vi "Red_Micro_Parse.vi"(10 "Data":string, 11 "String Array In":string[](array[string])) -> (2 "Redundant Micro out":T1, 3 "String Array Out":string[](array[string]))   [LabVIEW 2021]
uses:
  type defs/Redundant.ctl
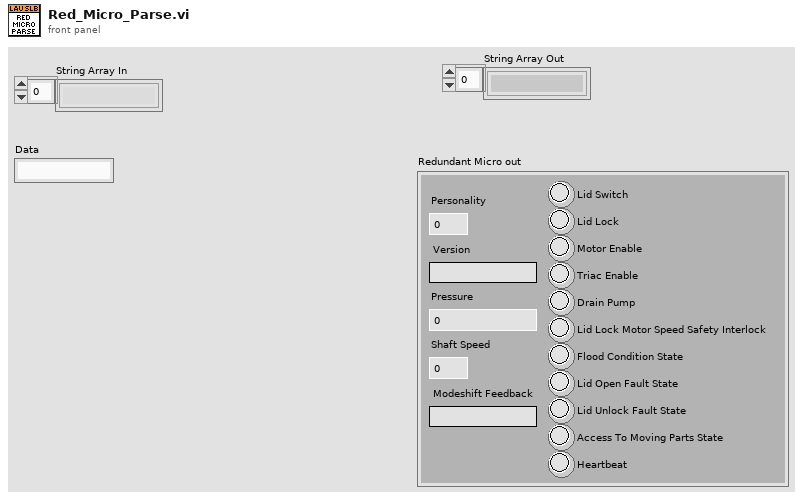
[diagram p1: front panel]
types:
  T1 = typedef "Redundant.ctl" = cluster{"Version":string, "Personality":u8, "Pressure ":dbl, "Shaft Speed":u16, "Modeshift Feedback":string, "Lid Switch":bool, "Lid Lock":bool, "Triac Enable":bool, "Drain Pump":bool, "Lid Lock Motor Speed Safety Interlock":bool, "Flood Condition State":bool, "Lid Open Fault State":bool, "Access To Moving Parts State":bool, "Heartbeat":bool, "Motor Enable":bool, "Lid Unlock Fault State":bool}
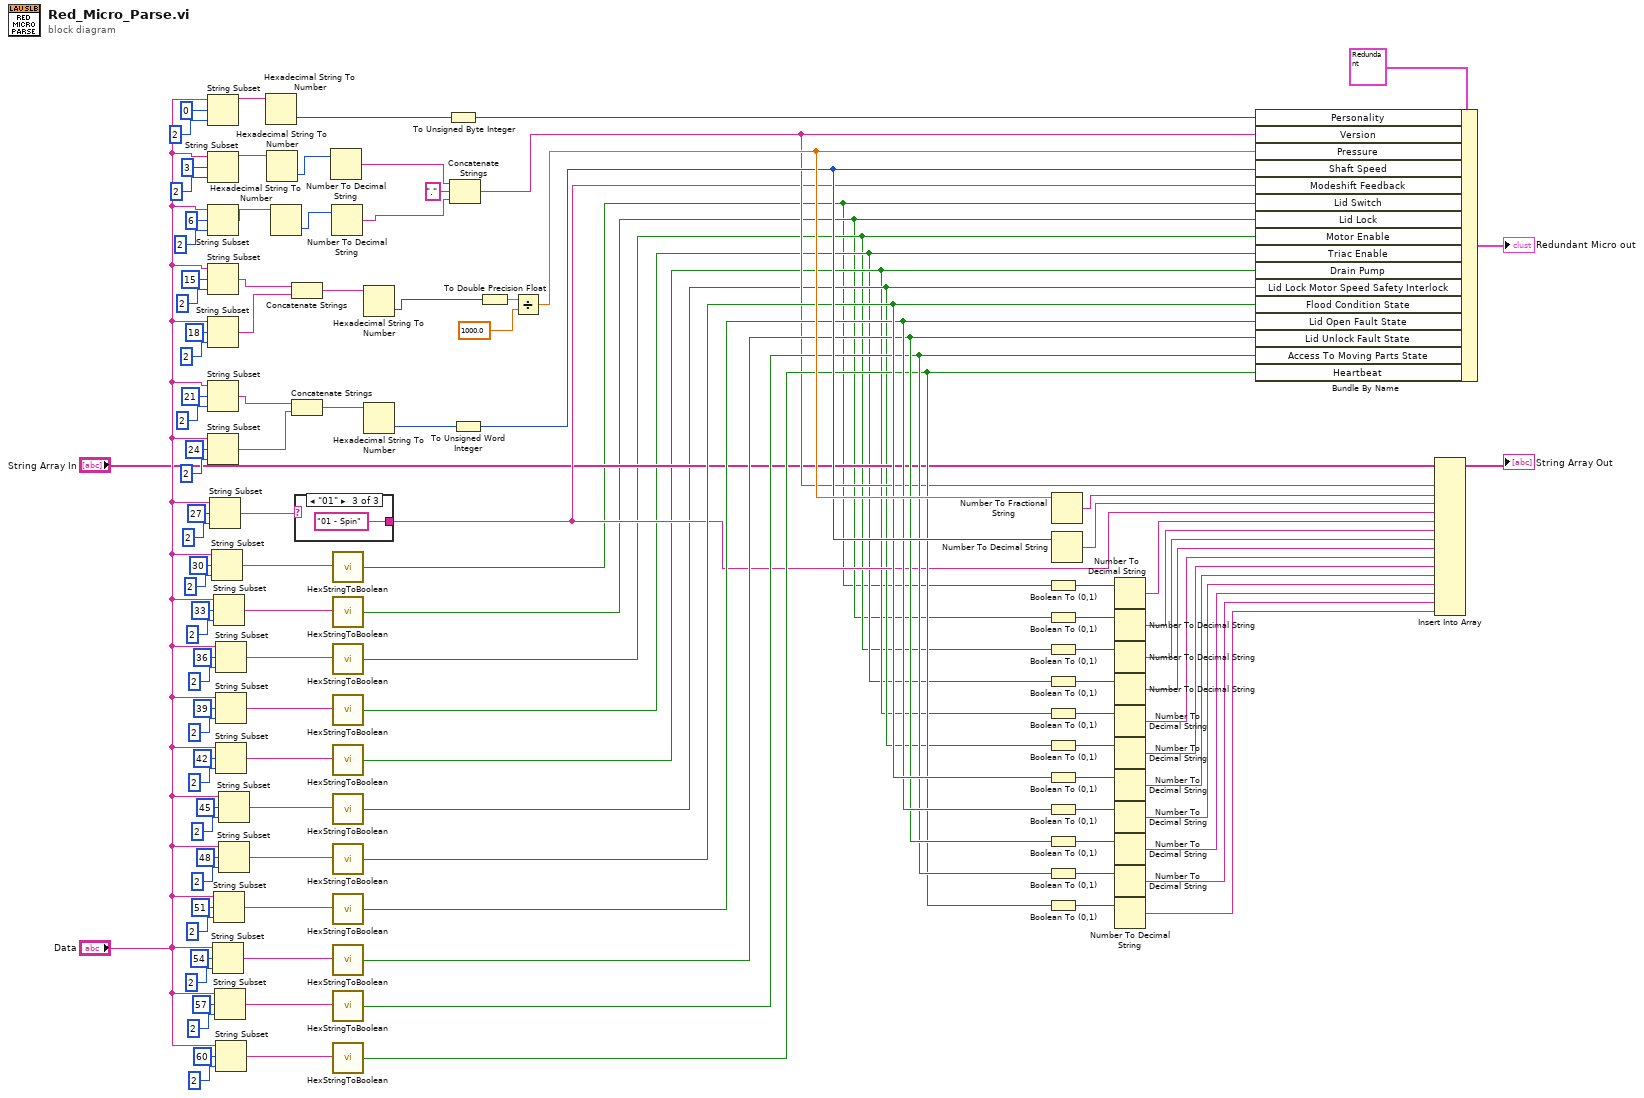
[diagram p0: block diagram]
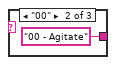
[diagram p3: hidden frame]
diagram:
  n1 = String Subset(string="Data", offset (0)=0, length (rest)=2 ("length (rest)")) -> (substring=w44:string)
  n2 = String Subset(string="Data", offset (0)=3, length (rest)=2 ("length (rest)")) -> (substring=w46:string)
  n3 = String Subset(string="Data", offset (0)=6, length (rest)=2 ("length (rest)")) -> (substring=w52:string)
  n4 = String Subset(string="Data", offset (0)=15, length (rest)=2 ("length (rest)")) -> (substring=w62:string)
  n5 = String Subset(string="Data", offset (0)=18, length (rest)=2 ("length (rest)")) -> (substring=w63:string)
  n6 = String Subset(string="Data", offset (0)=21, length (rest)=2 ("length (rest)")) -> (substring=w71:string)
  n7 = String Subset(string="Data", offset (0)=24, length (rest)=2 ("length (rest)")) -> (substring=w72:string)
  n8 = String Subset(string="Data", offset (0)=27, length (rest)=2 ("length (rest)")) -> (substring=w76:string)
  n9 = String Subset(string="Data", offset (0)=30, length (rest)=2 ("length (rest)")) -> (substring=w79:string)
  n10 = String Subset(string="Data", offset (0)=54, length (rest)=2 ("length (rest)")) -> (substring=w103:string)
  n11 = String Subset(string="Data", offset (0)=33, length (rest)=2 ("length (rest)")) -> (substring=w80:string)
  n12 = String Subset(string="Data", offset (0)=51, length (rest)=2 ("length (rest)")) -> (substring=w98:string)
  n13 = String Subset(string="Data", offset (0)=57, length (rest)=2 ("length (rest)")) -> (substring=w104:string)
  n14 = String Subset(string="Data", offset (0)=36, length (rest)=2 ("length (rest)")) -> (substring=w85:string)
  n15 = String Subset(string="Data", offset (0)=39, length (rest)=2 ("length (rest)")) -> (substring=w86:string)
  n16 = String Subset(string="Data", offset (0)=42, length (rest)=2 ("length (rest)")) -> (substring=w91:string)
  n17 = String Subset(string="Data", offset (0)=60, length (rest)=2 ("length (rest)")) -> (substring=w109:string)
  n18 = String Subset(string="Data", offset (0)=45, length (rest)=2 ("length (rest)")) -> (substring=w92:string)
  n19 = String Subset(string="Data", offset (0)=48, length (rest)=2 ("length (rest)")) -> (substring=w97:string)
  n20 = Hexadecimal String To Number(string=w44) -> (number=w45:u32)  [unwired: 2 in, 1 out]
  n21 = Hexadecimal String To Number(string=w46) -> (number=w53:u32)  [unwired: 2 in, 1 out]
  n22 = Hexadecimal String To Number(string=w52) -> (number=w54:u32)  [unwired: 2 in, 1 out]
  n23 = Concatenate Strings(w62, w63) -> (w64:string)
  n24 = Concatenate Strings(w71, w72) -> (w73:string)
  n25 = case shown="\"01\"" w76 {
    selector: w76 -> [w115 _ _]
    tunnel: [w115 "00 - Agitate" "01 - Spin"] -> w22
    frame Default {
    }
    frame "00" {
    }
    frame "01" {
    }
  }
  n26 = Number To Decimal String(number=w53) -> (decimal integer string=w57:string)  [unwired: 1 in]
  n27 = Number To Decimal String(number=w54) -> (decimal integer string=w56:string)  [unwired: 1 in]
  n28 = call "HexStringToBoolean.vi"("Hex String"=w79) -> ("Boolean"=w2:bool)
  n29 = call "HexStringToBoolean.vi"("Hex String"=w80) -> ("Boolean"=w3:bool)
  n30 = call "HexStringToBoolean.vi"("Hex String"=w85) -> ("Boolean"=w4:bool)
  n31 = call "HexStringToBoolean.vi"("Hex String"=w86) -> ("Boolean"=w5:bool)
  n32 = call "HexStringToBoolean.vi"("Hex String"=w91) -> ("Boolean"=w6:bool)
  n33 = call "HexStringToBoolean.vi"("Hex String"=w92) -> ("Boolean"=w7:bool)
  n34 = call "HexStringToBoolean.vi"("Hex String"=w97) -> ("Boolean"=w28:bool)
  n35 = call "HexStringToBoolean.vi"("Hex String"=w98) -> ("Boolean"=w27:bool)
  n36 = call "HexStringToBoolean.vi"("Hex String"=w103) -> ("Boolean"=w26:bool)
  n37 = call "HexStringToBoolean.vi"("Hex String"=w104) -> ("Boolean"=w25:bool)
  n38 = call "HexStringToBoolean.vi"("Hex String"=w109) -> ("Boolean"=w24:bool)
  n39 = Hexadecimal String To Number(string=w64) -> (number=w65:u32)  [unwired: 2 in, 1 out]
  n40 = Hexadecimal String To Number(string=w73) -> (number=w66:u32)  [unwired: 2 in, 1 out]
  n41 = To Unsigned Byte Integer(number=w45) -> (unsigned 8bit integer=w49:u8)
  n42 = Concatenate Strings(w57, "." ("string"), w56) -> (w23:string)
  n43 = To Unsigned Word Integer(number=w66) -> (unsigned 16bit integer=w29:u16)
  n44 = To Double Precision Float(number=w65) -> (double precision float=w110:dbl)
  n45 = Divide(x=w110, y=1000.0) -> (x/y=w30:dbl)
  n46 = Boolean To (0,1)(Boolean=w2) -> (0, 1=w41:i16)
  n47 = Boolean To (0,1)(Boolean=w3) -> (0, 1=w40:i16)
  n48 = Boolean To (0,1)(Boolean=w4) -> (0, 1=w39:i16)
  n49 = Boolean To (0,1)(Boolean=w5) -> (0, 1=w38:i16)
  n50 = Boolean To (0,1)(Boolean=w6) -> (0, 1=w37:i16)
  n51 = Boolean To (0,1)(Boolean=w7) -> (0, 1=w36:i16)
  n52 = Boolean To (0,1)(Boolean=w28) -> (0, 1=w35:i16)
  n53 = Boolean To (0,1)(Boolean=w27) -> (0, 1=w34:i16)
  n54 = Boolean To (0,1)(Boolean=w26) -> (0, 1=w33:i16)
  n55 = Boolean To (0,1)(Boolean=w25) -> (0, 1=w32:i16)
  n56 = Boolean To (0,1)(Boolean=w24) -> (0, 1=w31:i16)
  n57 = Number To Fractional String(number=w30) -> (F-format string=w21:string)  [unwired: 3 in]
  n58 = Number To Decimal String(number=w29) -> (decimal integer string=w20:string)  [unwired: 1 in]
  n59 = Number To Decimal String(number=w41) -> (decimal integer string=w19:string)  [unwired: 1 in]
  n60 = Number To Decimal String(number=w40) -> (decimal integer string=w18:string)  [unwired: 1 in]
  n61 = Number To Decimal String(number=w39) -> (decimal integer string=w17:string)  [unwired: 1 in]
  n62 = Number To Decimal String(number=w38) -> (decimal integer string=w16:string)  [unwired: 1 in]
  n63 = Number To Decimal String(number=w37) -> (decimal integer string=w15:string)  [unwired: 1 in]
  n64 = Number To Decimal String(number=w36) -> (decimal integer string=w14:string)  [unwired: 1 in]
  n65 = Number To Decimal String(number=w35) -> (decimal integer string=w13:string)  [unwired: 1 in]
  n66 = Number To Decimal String(number=w34) -> (decimal integer string=w12:string)  [unwired: 1 in]
  n67 = Number To Decimal String(number=w33) -> (decimal integer string=w11:string)  [unwired: 1 in]
  n68 = Number To Decimal String(number=w32) -> (decimal integer string=w10:string)  [unwired: 1 in]
  n69 = Number To Decimal String(number=w31) -> (decimal integer string=w9:string)  [unwired: 1 in]
  n70 = Bundle By Name(cluster=T1 {"Version"="", "Personality"=0, "Pressure "=0.0, "Shaft Speed"=0, "Modeshift Feedback"="", "Lid Switch"=FALSE, "Lid Lock"=FALSE, "Triac Enable"=FALSE, "Drain Pump"=FALSE, "Lid Lock Motor Speed Safety Interlock"=FALSE, "Flood Condition State"=FALSE, "Lid Open Fault State"=FALSE, "Access To Moving Parts State"=FALSE, "Heartbeat"=FALSE, "Motor Enable"=FALSE, "Lid Unlock Fault State"=FALSE} ("Redundant Micro in"), "Personality"=w49, "Version"=w23, "Pressure"=w30, "Shaft Speed"=w29, "Modeshift Feedback"=w22, "Lid Switch"=w2, "Lid Lock"=w3, "Motor Enable"=w4, "Triac Enable"=w5, "Drain Pump"=w6, "Lid Lock Motor Speed Safety Interlock"=w7, "Flood Condition State"=w28, "Lid Open Fault State"=w27, "Lid Unlock Fault State"=w26, "Access To Moving Parts State"=w25, "Heartbeat"=w24) -> (→"Redundant Micro out":T1)
  n71 = Insert Into Array(array="String Array In", new element #1=w23, new element #2=w21, new element #3=w20, new element #4=w22, new element #5=w19, new element #6=w18, new element #7=w17, new element #8=w16, new element #9=w15, new element #10=w14, new element #11=w13, new element #12=w12, new element #13=w11, new element #14=w10, new element #15=w9) -> (→"String Array Out":string[])  [unwired: 1 in]
